vi "Subvi address gen.vi"(4 "Line gating":bool, 9 "Gated pixel clock":bool) -> ()   [LabVIEW 2017]
uses:
  <vilib>/rvi/Emulation/niFpgaSctlEmulationGetInTimedLoop.vi
  Probes/GV DO5.vi
  <vilib>/rvi/Emulation/niFpgaProcessEmulError.vi
  GV memory address.vi
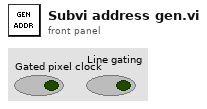
[diagram p1: front panel]
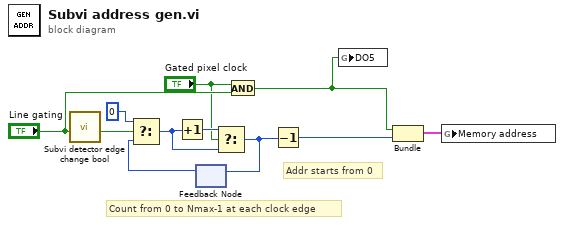
[diagram p0: block diagram]
diagram:
  # "Addr starts from 0"
  # "Count from 0 to Nmax-1 at each clock edge"
  n1 = call "Subvi detector edge change bool.vi"("Input"="Line gating") -> ("Output"=w6:bool)  [unwired: 8 in]
  n2 = feedback #1() -> (w8:u16)  [unwired: 1 in]
  n3 = Select(t=u16 0, s=w6, f=w8) -> (s? t:f=w9:u16)
  n4 = Increment(x=w9) -> (x+1=w10:u16)
  n5 = Select(t=w10, s="Gated pixel clock", f=w9) -> (s? t:f=w11:u16)
  n6 = feedback-in #1(w11) -> ()
  n7 = And(x="Gated pixel clock", y="Line gating") -> (x .and. y?=w1:bool)
  n8 = Decrement(x=w11) -> (x-1=w2:u16)
  n9 = global write "GV DO5.vi" "DO5"(w1) -> ()
  n10 = Bundle(w1, w2) -> (w3:cluster{bool, u16})  [unwired: 1 in]
  n11 = global write "GV memory address.vi" "Memory address"(w3) -> ()
